vi "add y_column names.vi"(9 "column extension":string[](array[string])=["100", "101", "102"], 10 "old y-column names":string[](array[string]), 11 "graph file":cluster{"all rows":dbl[], "all rows":dbl[]}[](array[cluster])=[{"all rows"=[0.0, 1.0], "all rows"=[0.0, 1.0]}, {"all rows"=[0.0, 1.0], "all rows"=[0.0, 1.0]}] {"all rows" format="%.2e"; "all rows" format="%.2f"}) -> (0 "col extension size":i32, 1 "new y-column names size":i32, 3 "new y-column names":string[](array[string]))   [LabVIEW 2024]
panel:
  out "# of plots":i32
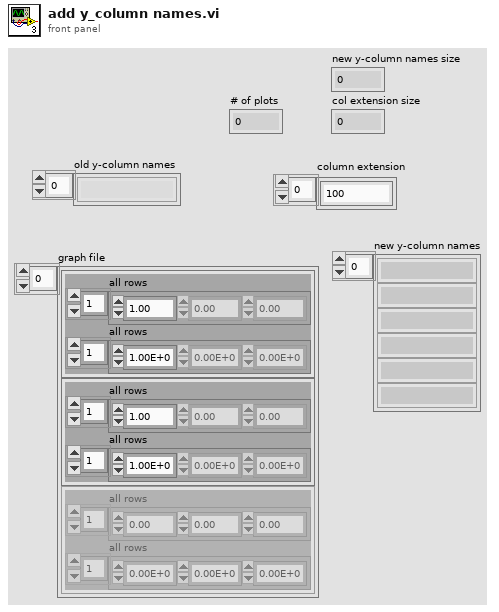
[diagram p1: front panel]
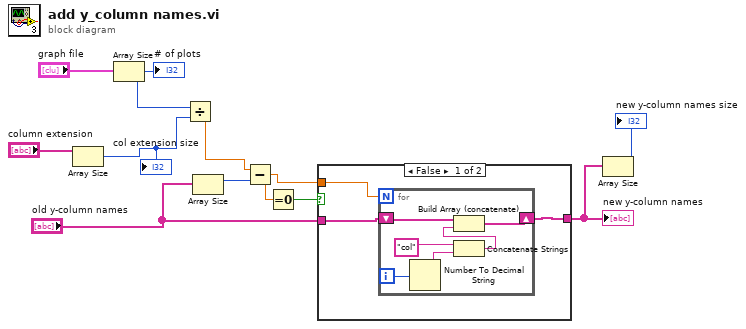
[diagram p0: block diagram]
diagram:
  n1 = Array Size(array="column extension") -> (size(s)=w4:i32)
  "col extension size" <- w4
  n2 = Array Size(array="graph file") -> (size(s)=w6:i32)
  "# of plots" <- w6
  n3 = Divide(x=w6, y=w4) -> (x/y=w3:dbl)
  n4 = Array Size(array="old y-column names") -> (size(s)=w8:i32)
  n5 = Subtract(x=w3, y=w8) -> (x-y=w11:dbl)
  n6 = Equal To 0?(x=w11) -> (x = 0?=w9:bool)
  n7 = case shown="False" w9 {
    tunnel: "old y-column names" -> [w12 w21]
    tunnel: [w13 w21] -> w2
    tunnel: w11 -> [w14 _]
    frame False {
      n8 = for {
        N: w14 -> [_]
        shift-right: [w16] -> w13
        shift-left: w12 -> [w17]
        i -> [w20]
        n9 = Number To Decimal String(number=w20) -> (decimal integer string=w18:string)  [unwired: 1 in]
        n10 = Concatenate Strings("col", w18) -> (w15:string)
        n11 = Build Array (concatenate)(w17, w15) -> (w16:string[])
      }
    }
    frame True {
    }
  }
  "new y-column names" <- w2
  n12 = Array Size(array=w2) -> (size(s)=→"new y-column names size":i32)
